vi "Main.vi"(8 "error in":errorcluster, 11 "TCP Server Example in":refnum<class "TCP Server Example.lvclass">) -> (0 "error out":errorcluster, 3 "TCP Server Example out":refnum<class "TCP Server Example.lvclass">)   [LabVIEW 2017, in "TCP Server Example.lvclass"]
doc: "The <b>Queued Message Handler</b> of the Worker that owns this VI."
uses:
  TCP Server Example.lvclass
  C:/SC/Source Code/VIPM/LabVIEW 20xx/vi.lib/addons/_Workers/Library/Classes/Worker/Worker.lvclass
  Client Data.ctl
  TCP Server Example.lvclass/TCP Server Example.ctl
  Initialization Data.ctl
  TCP Server/TCP Server/rqp_Start Listening.ctl
  TCP Server/TCP Server/rqp_Send String to Clients.ctl
  TCP Server/TCP Server/rqp_Disconnect Clients.ctl
  <vilib>/addons/_Workers/Library/Classes/Message Queue/Message Queue.lvclass
  TCP Server/TCP Server/TCP Server.lvclass
panel:
  in  "Server Name":string="TCP Server"
  out "Listening":bool
  in  "Server Port":u16=7654
  in  "Start/Stop Listening":bool caption="Disconnect from Server"
  in  "Client 2":T1
  out "Title":string="TCP Server Example"
  in  "Client 1":T1
  # "Server Name"
  # "Server Port"
  # "( 1 : N connections )"
  # "The Workers TCP Server can accept connections from multiple TCP Clients. This example shows how one TCP Server can be connected to two TCP Clients."
  # "Client Name :"
  # "IP Address :"
  # "Connected? :"
  # "Client Name :"
  # "IP Address :"
  # "Connected? :"
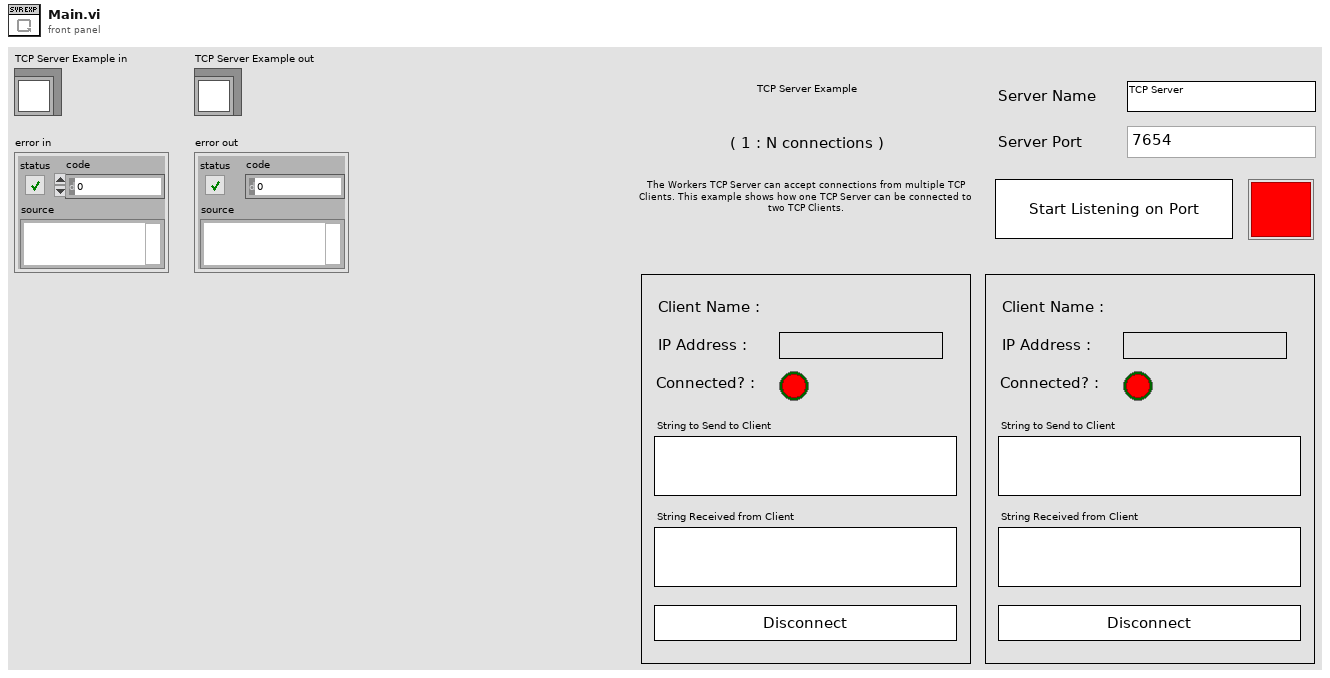
[diagram p1: front panel]
types:
  T1 = typedef "TCP Server Example.lvclass/Client Data.ctl" = cluster{"Client Name":string, "IP Address":string, "Connected?":bool, "String to Send to Client":string, "String Received from Client":string, "Disconnect from Client":bool}
  T2 = typedef "TCP Server Example.lvclass/Initialization Data.ctl" = cluster{"String":string}
  T3 = typedef "_TCP Server.lvlib/TCP Server.lvclass/rqp_Start Listening.ctl" = cluster{"Server Name":string, "Server IP Address":string, "Server Port":u16}
  T4 = typedef "_TCP Server.lvlib/TCP Server.lvclass/rqp_Send String to Clients.ctl" = cluster{"TCP Client Names":string[], "String to Send":string}
  T5 = typedef "_TCP Server.lvlib/TCP Server.lvclass/rqp_Disconnect Clients.ctl" = cluster{"TCP Client Names":string[]}
  T6 = typedef "_TCP Server.lvlib/TCP Server.lvclass/rsp_Connection Notify.ctl" = cluster{"Client Name":string, "IP Address":string, "Connected?":bool}
  T7 = typedef "_TCP Server.lvlib/TCP Server.lvclass/rsp_Incoming Data.ctl" = cluster{"Client Name":string, "Data":string}
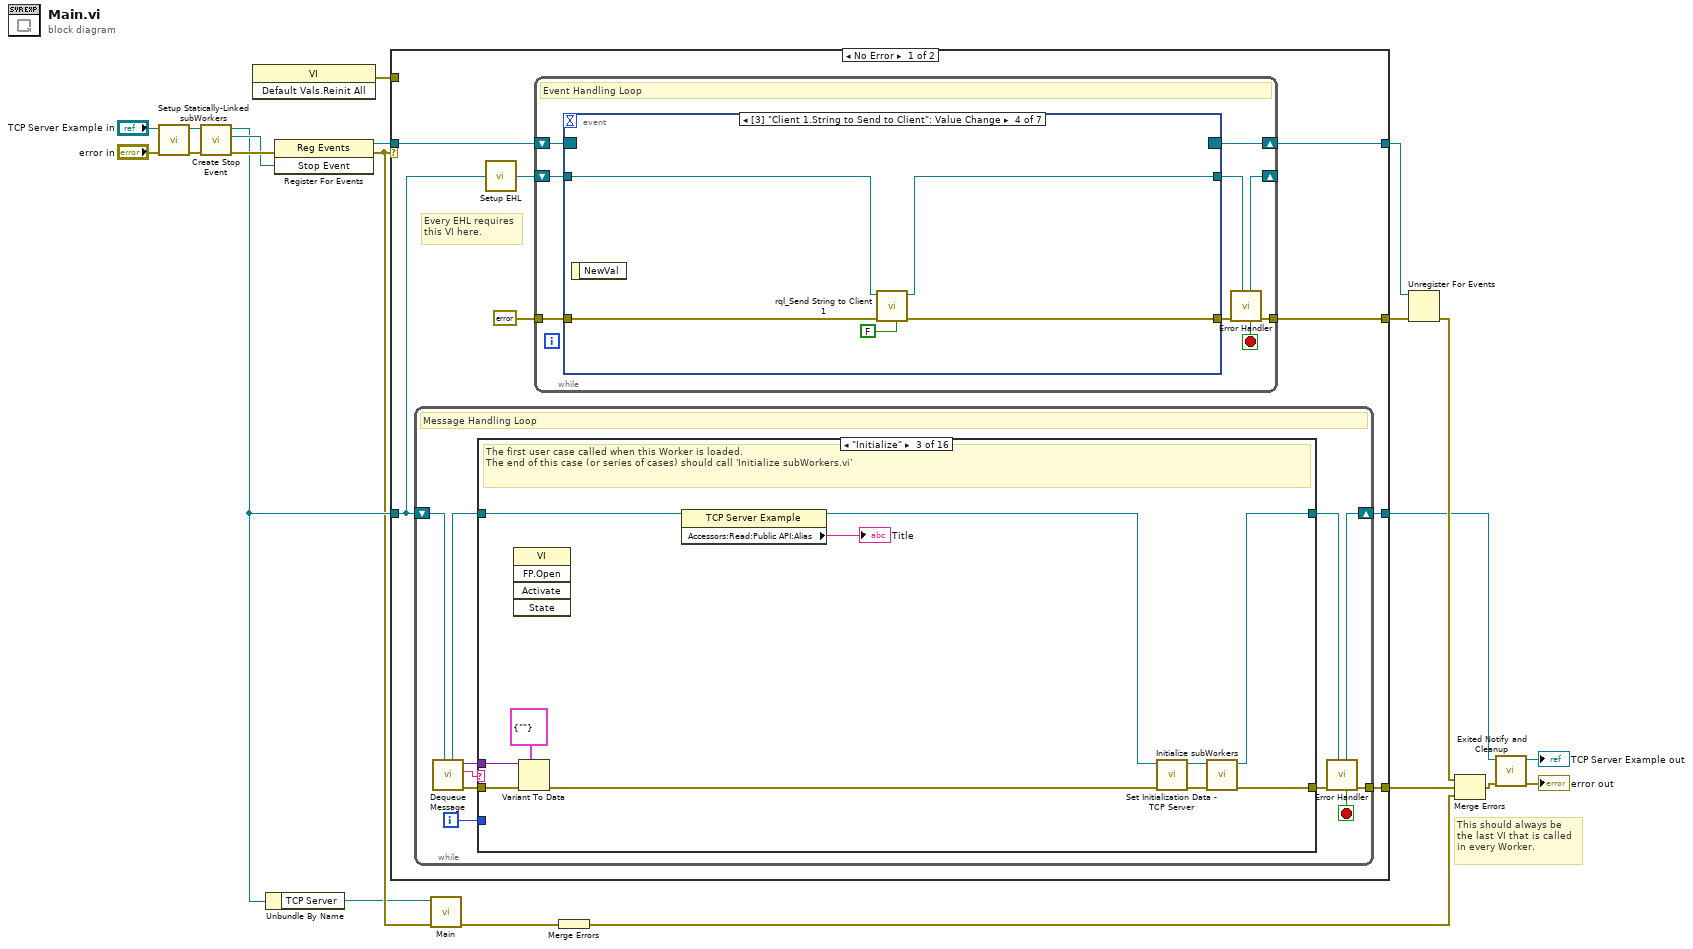
[diagram p0: block diagram]
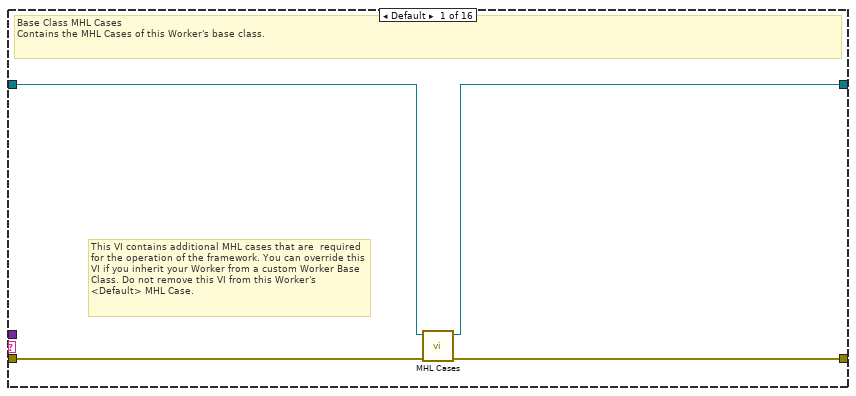
[diagram p2: hidden frame]
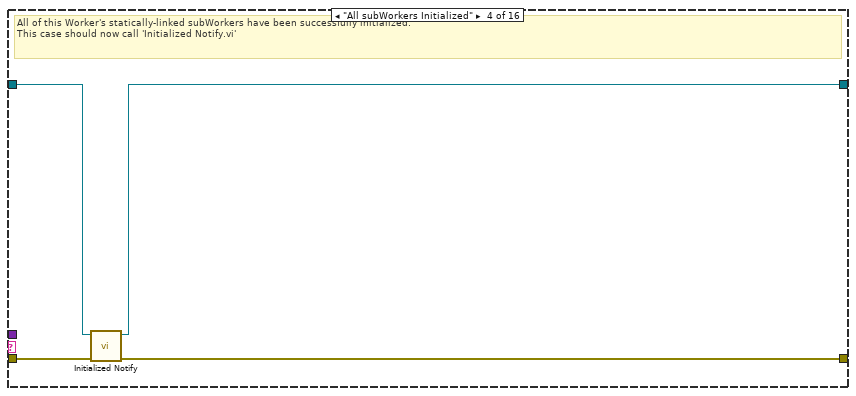
[diagram p4: hidden frame]
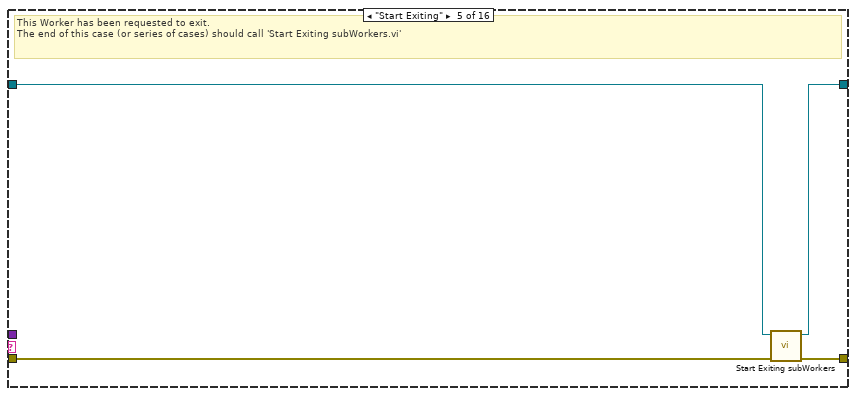
[diagram p5: hidden frame]
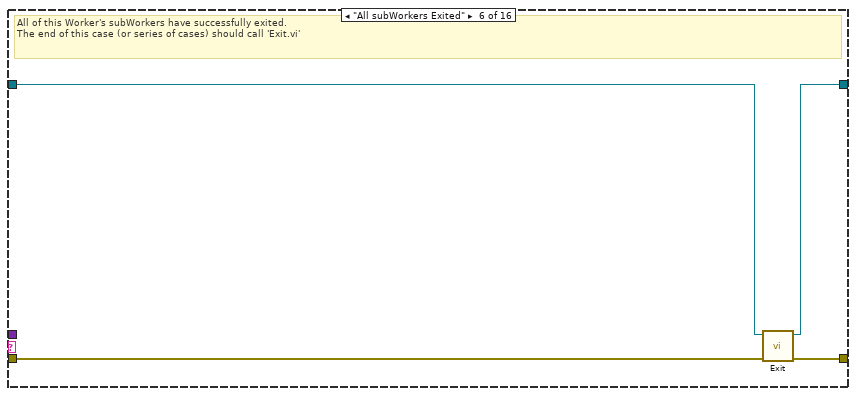
[diagram p6: hidden frame]
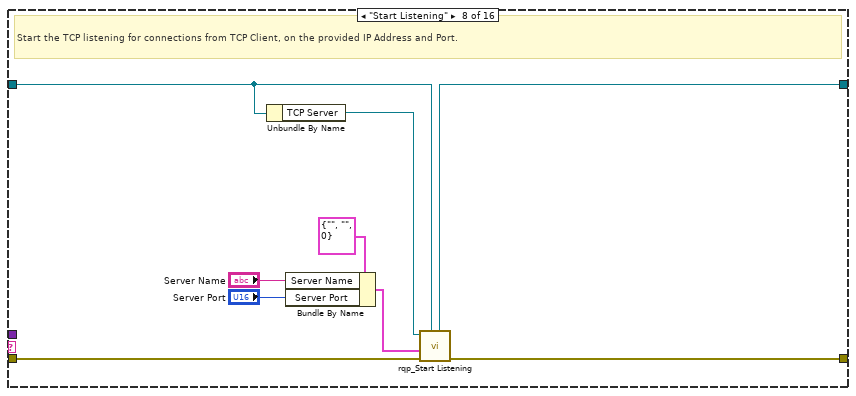
[diagram p8: hidden frame]
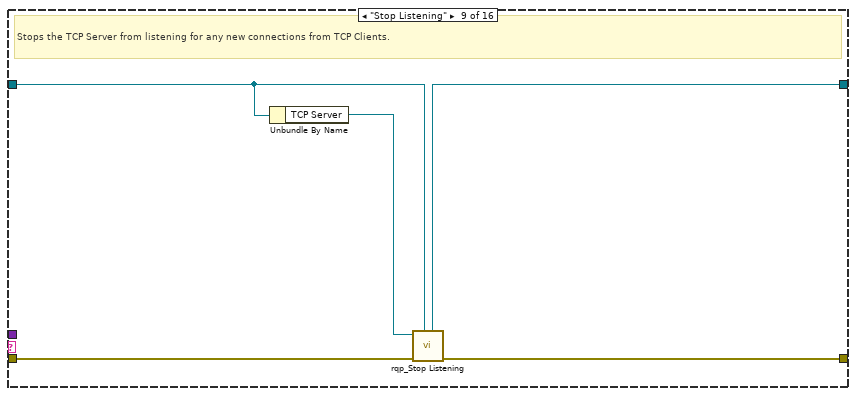
[diagram p9: hidden frame]
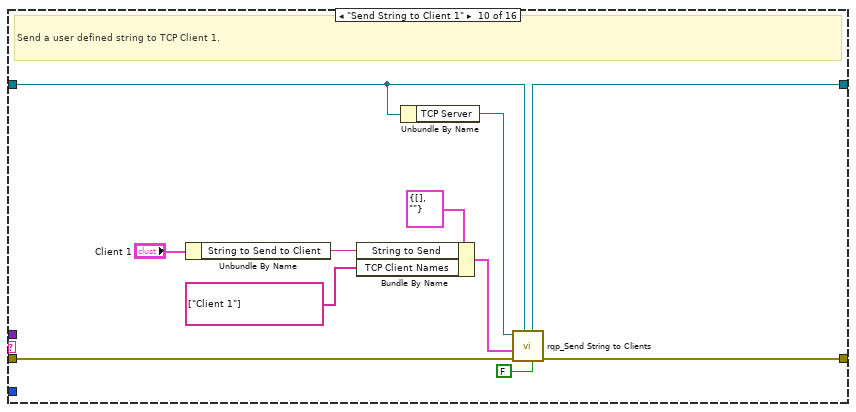
[diagram p10: hidden frame]
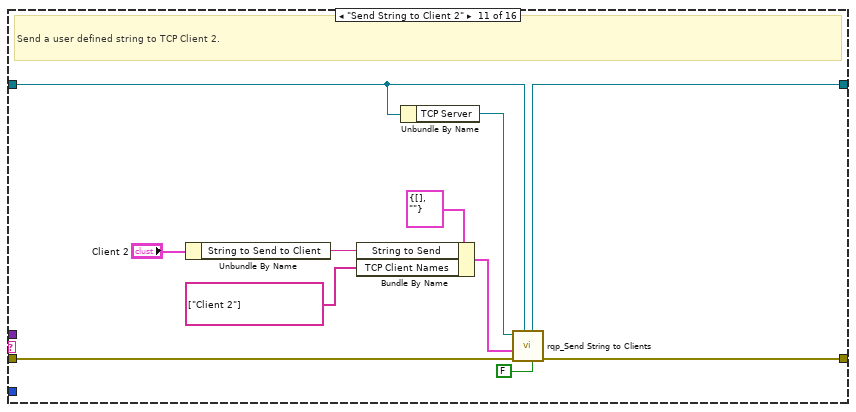
[diagram p11: hidden frame]
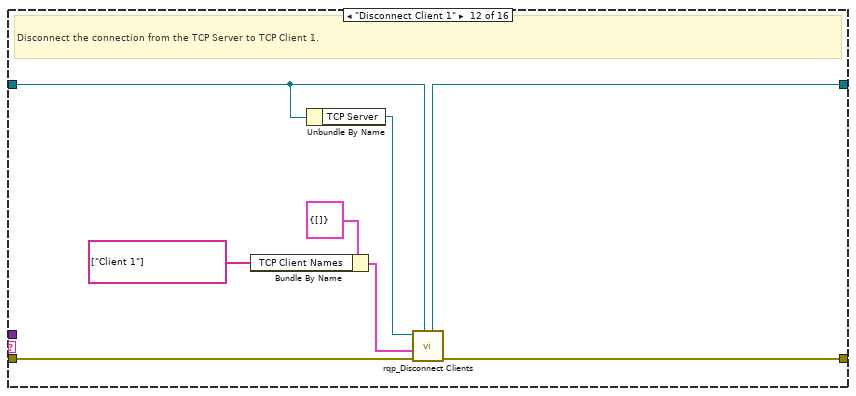
[diagram p12: hidden frame]
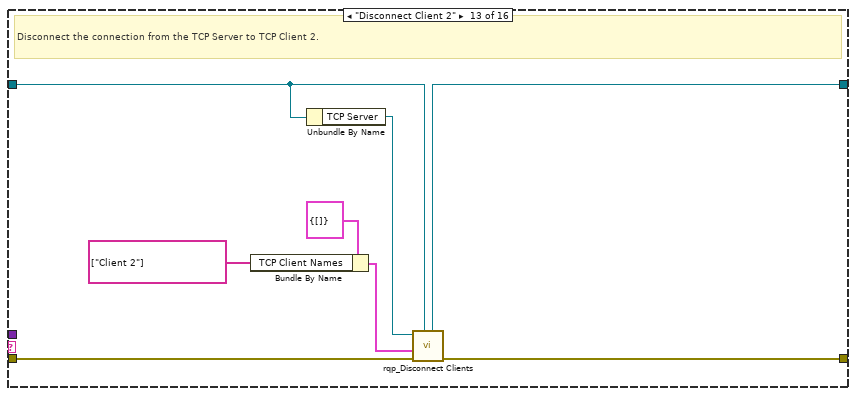
[diagram p13: hidden frame]
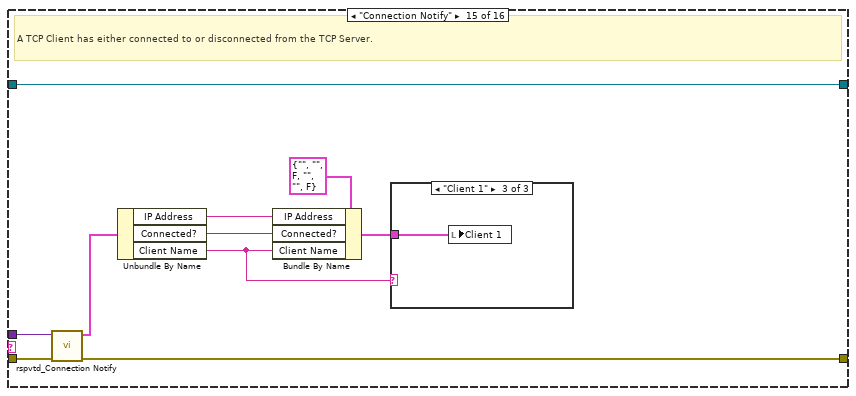
[diagram p15: hidden frame]
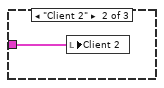
[diagram p17: hidden frame]
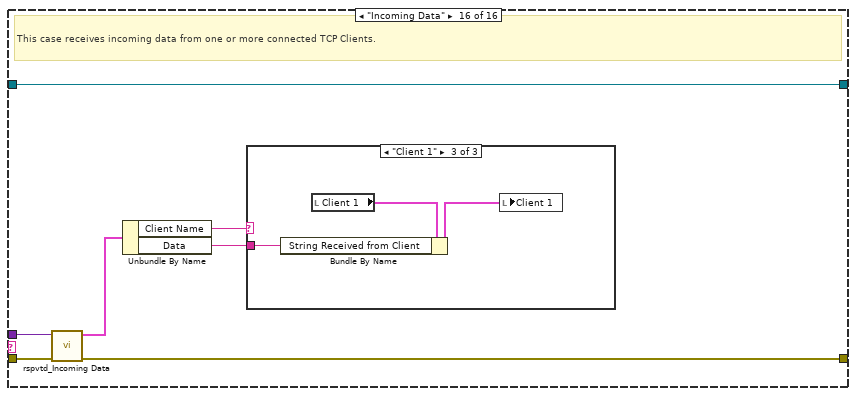
[diagram p18: hidden frame]
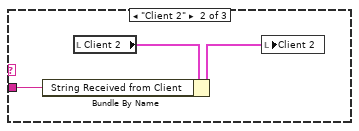
[diagram p20: hidden frame]
diagram:
  # "This should always be the last VI that is called in every Worker."
  n1 = call "Setup Statically-Linked subWorkers.vi"("error in"="error in", "TCP Server Example in"="TCP Server Example in") -> ("error out"=w6:errorcluster, "TCP Server Example out"=w4:refnum<class "TCP Server Example.lvclass">)  [unwired: 8 in]
  n2 = call-dynamic "Create Stop Event.vi"("error in"=w6, "Worker"=w4) -> ("error out"=w16:errorcluster, "Stop Event"=w13:refnum<user-event>, "Worker out"=w10:refnum<class "TCP Server Example.lvclass">)  [unwired: 7 in]
  n3 = invoke class="VI" method="Default Vals.Reinit All"() -> (error out=w8:errorcluster)  [unwired: 3 in, 2 out]
  n4 = Unbundle By Name(w10) -> ("TCP Server"=w1:refnum<class "TCP Server.lvclass">)
  n5 = register-events(error in=w16, w13) -> (reference out=w15:refnum<event-registration>, error out=w9:errorcluster)  [unwired: 1 in]
  n6 = case shown="No Error" w9 {
    tunnel: w10 -> [w24 w211]
    tunnel: [w22 w212] -> w14
    tunnel: w15 -> [w29 w213]
    tunnel: [w26 w214] -> w20
    tunnel: [w28 w213] -> w19
    tunnel: [w23 w210] -> w17
    selector: w9 -> [_ w214]
    tunnel: w8 -> [_ _]
    frame No Error {
      # "Every EHL requires\nthis VI here."
      n7 = while {
        shift-right: [w38] -> w23
        shift-left: w24 -> [w40]
        tunnel: [w39] -> w22
        i -> [w31]
        stop <- w32 stop-if-true
        # "Message Handling Loop"
        n8 = call-dynamic "Dequeue Message.vi"("Worker"=w40) -> ("error out"=w37:errorcluster, "Case out"=w33:string, "Data out"=w30:variant, "Worker out"=w35:refnum<class "TCP Server Example.lvclass">)  [unwired: 6 in, 1 out]
        n9 = case "Worker MHL Case Structure (DO NOT CHANGE LABEL NAME)" shown="\"Initialize\"" w33 {
          tunnel: w37 -> [w44 w45 w55 w60 w62 w69 w71 w80 w85 w96 w107 w115 w123 w125 w135 w144]
          tunnel: [w43 w45 w57 w58 w65 w68 w71 w79 w84 w95 w106 w114 w122 w125 w133 w142] -> w36
          tunnel: w35 -> [w42 w46 w52 w61 w63 w67 w70 w73 w82 w92 w104 w112 w120 w124 w134 w143]
          tunnel: [w41 w46 w56 w59 w64 w66 w70 w78 w83 w94 w105 w113 w121 w124 w134 w143] -> w34
          tunnel: w31 -> [_ _ _ _ _ _ _ _ _ _ _ _ _ _ _ _]
          tunnel: w30 -> [_ _ w53 _ _ _ _ _ _ _ _ _ _ _ w132 w141]
          frame Default {
            # "This VI contains additional MHL cases that are  required for the operation of the framework. You can override this VI if you inherit your Worker from a custom Worker Base Class. Do not remove this VI from this Worker's <Default> MHL Case."
            # "Base Class MHL Cases\nContains the MHL Cases of this Worker's base class."
            n10 = call-dynamic "MHL Cases.vi"("error in"=w44, "Worker in"=w42) -> ("error out"=w43:errorcluster, "Worker out"=w41:refnum<class "TCP Server Example.lvclass">)  [unwired: 8 in]
          }
          frame "------------ FRAMEWORK CASES -----------" {
            # "Start of Workers Framework Cases"
          }
          frame "Initialize" {
            # "The first user case called when this Worker is loaded.\nThe end of this case (or series of cases) should call 'Initialize subWorkers.vi'"
            n11 = invoke class="VI" method="FP.Open"() -> ()  [unwired: 5 in, 5 out]
            n12 = Variant To Data(error in=w55, type=T2 {"String"=""} ("Initialization Data"), Variant=w53) -> (error out=w54:errorcluster)  [unwired: 1 out]
            n13 = property class="TCP Server Example"(reference=w52) -> (reference out=w47:refnum<class "TCP Server Example.lvclass">, "Accessors:Read:Public API:Alias"=→"Title":string)  [unwired: 1 in, 1 out]
            n14 = call "Set Initialization Data - TCP Server.vi"("error in"=w54, "TCP Server Example in"=w47) -> ("error out"=w49:errorcluster, "TCP Server Example out"=w48:refnum<class "TCP Server Example.lvclass">)  [unwired: 8 in]
            n15 = call-dynamic "Initialize subWorkers.vi"("error in"=w49, "Worker"=w48) -> ("error out"=w57:errorcluster, "dup Worker out"=w56:refnum<class "TCP Server Example.lvclass">)  [unwired: 8 in]
          }
          frame "All subWorkers Initialized" {
            # "All of this Worker's statically-linked subWorkers have been successfully initialized.\nThis case should now call 'Initialized Notify.vi'"
            n16 = call-dynamic "Initialized Notify.vi"("error in"=w60, "Worker"=w61) -> ("error out"=w58:errorcluster, "dup Worker out"=w59:refnum<class "TCP Server Example.lvclass">)  [unwired: 8 in]
          }
          frame "Start Exiting" {
            # "This Worker has been requested to exit. \nThe end of this case (or series of cases) should call 'Start Exiting subWorkers.vi'"
            n17 = call-dynamic "Start Exiting subWorkers.vi"("error_in"=w62, "Worker"=w63) -> ("error out"=w65:errorcluster, "dup Worker out"=w64:refnum<class "TCP Server Example.lvclass">)  [unwired: 8 in]
          }
          frame "All subWorkers Exited" {
            # "All of this Worker's subWorkers have successfully exited. \nThe end of this case (or series of cases) should call 'Exit.vi'"
            n18 = call-dynamic "Exit.vi"("error_in"=w69, "Worker"=w67) -> ("error out"=w68:errorcluster, "dup Worker out"=w66:refnum<class "TCP Server Example.lvclass">)  [unwired: 8 in]
          }
          frame "------------- LOCAL API CASES -------------" {
            # "Start of Workers Local API Cases"
          }
          frame "Start Listening" {
            # "Start the TCP listening for connections from TCP Client, on the provided IP Address and Port."
            n19 = Unbundle By Name(w73) -> ("TCP Server"=w72:refnum<class "TCP Server.lvclass">)
            n20 = Bundle By Name(cluster=T3 {"Server Name"="", "Server IP Address"="", "Server Port"=0} ("Data"), "Server Name"="Server Name", "Server Port"="Server Port") -> (w76:T3)
            n21 = call "rqp_Start Listening.vi"("Caller in"=w73, "error in"=w80, "Data in"=w76, "TCP Server in"=w72) -> ("error out"=w79:errorcluster, "dup Caller out"=w78:refnum<class "TCP Server Example.lvclass">)  [unwired: 5 in, 1 out]
          }
          frame "Stop Listening" {
            # "Stops the TCP Server from listening for any new connections from TCP Clients."
            n22 = Unbundle By Name(w82) -> ("TCP Server"=w81:refnum<class "TCP Server.lvclass">)
            n23 = call "rqp_Stop Listening.vi"("Caller in"=w82, "error in"=w85, "TCP Server in"=w81) -> ("error out"=w84:errorcluster, "dup Caller out"=w83:refnum<class "TCP Server Example.lvclass">)  [unwired: 6 in, 1 out]
          }
          frame "Send String to Client 1" {
            # "Send a user defined string to TCP Client 1."
            n24 = Unbundle By Name("Client 1") -> ("String to Send to Client"=w88:string)
            n25 = Bundle By Name(cluster=T4 {"TCP Client Names"=[], "String to Send"=""} ("Data in"), "String to Send"=w88, "TCP Client Names"=string[] ["Client 1"]) -> (w89:T4)
            n26 = Unbundle By Name(w92) -> ("TCP Server"=w91:refnum<class "TCP Server.lvclass">)
            n27 = call "rqp_Send String to Clients.vi"("Show in Debugger?"=FALSE, "Caller in"=w92, "error in"=w96, "Data in"=w89, "TCP Server in"=w91) -> ("error out"=w95:errorcluster, "dup Caller out"=w94:refnum<class "TCP Server Example.lvclass">)  [unwired: 4 in, 1 out]
          }
          frame "Send String to Client 2" {
            # "Send a user defined string to TCP Client 2."
            n28 = Unbundle By Name("Client 2") -> ("String to Send to Client"=w100:string)
            n29 = Bundle By Name(cluster=T4 {"TCP Client Names"=[], "String to Send"=""} ("Data in"), "String to Send"=w100, "TCP Client Names"=string[] ["Client 2"]) -> (w101:T4)
            n30 = Unbundle By Name(w104) -> ("TCP Server"=w103:refnum<class "TCP Server.lvclass">)
            n31 = call "rqp_Send String to Clients.vi"("Show in Debugger?"=FALSE, "Caller in"=w104, "error in"=w107, "Data in"=w101, "TCP Server in"=w103) -> ("error out"=w106:errorcluster, "dup Caller out"=w105:refnum<class "TCP Server Example.lvclass">)  [unwired: 4 in, 1 out]
          }
          frame "Disconnect Client 1" {
            # "Disconnect the connection from the TCP Server to TCP Client 1."
            n32 = Bundle By Name(cluster=T5 {"TCP Client Names"=[]} ("Data in"), "TCP Client Names"=string[] ["Client 1"]) -> (w109:T5)
            n33 = Unbundle By Name(w112) -> ("TCP Server"=w111:refnum<class "TCP Server.lvclass">)
            n34 = call "rqp_Disconnect Clients.vi"("Caller in"=w112, "error in"=w115, "Data in"=w109, "TCP Server in"=w111) -> ("error out"=w114:errorcluster, "dup Caller out"=w113:refnum<class "TCP Server Example.lvclass">)  [unwired: 5 in, 1 out]
          }
          frame "Disconnect Client 2" {
            # "Disconnect the connection from the TCP Server to TCP Client 2."
            n35 = Bundle By Name(cluster=T5 {"TCP Client Names"=[]} ("Data in"), "TCP Client Names"=string[] ["Client 2"]) -> (w117:T5)
            n36 = Unbundle By Name(w120) -> ("TCP Server"=w119:refnum<class "TCP Server.lvclass">)
            n37 = call "rqp_Disconnect Clients.vi"("Caller in"=w120, "error in"=w123, "Data in"=w117, "TCP Server in"=w119) -> ("error out"=w122:errorcluster, "dup Caller out"=w121:refnum<class "TCP Server Example.lvclass">)  [unwired: 5 in, 1 out]
          }
          frame "------------- RESPONSE CASES --------------" {
            # "Start of Workers Response Cases"
          }
          frame "Connection Notify" {
            # "A TCP Client has either connected to or disconnected from the TCP Server."
            n38 = call "rspvtd_Connection Notify.vi"("error in"=w135, "Data in"=w132) -> ("error out"=w133:errorcluster, "Data out"=w131:T6)  [unwired: 8 in]
            n39 = Unbundle By Name(w131) -> ("IP Address"=w128:string, "Connected?"=w129:bool, "Client Name"=w127:string)
            n40 = Bundle By Name(cluster=T1 {"Client Name"="", "IP Address"="", "Connected?"=FALSE, "String to Send to Client"="", "String Received from Client"="", "Disconnect from Client"=FALSE} ("Client Connection 1"), "IP Address"=w128, "Connected?"=w129, "Client Name"=w127) -> (w126:T1)
            n41 = case shown="\"Client 1\"" w127 {
              tunnel: w126 -> [_ w136 w137]
              frame Default {
              }
              frame "Client 2" {
                n42 = local write "Client 2"(w136) -> ()
              }
              frame "Client 1" {
                n43 = local write "Client 1"(w137) -> ()
              }
            }
          }
          frame "Incoming Data" {
            # "This case receives incoming data from one or more connected TCP Clients."
            n44 = call "rspvtd_Incoming Data.vi"("error in"=w144, "Data in"=w141) -> ("error out"=w142:errorcluster, "Data out"=w140:T7)  [unwired: 8 in]
            n45 = Unbundle By Name(w140) -> ("Client Name"=w139:string, "Data"=w138:string)
            n46 = case shown="\"Client 1\"" w139 {
              tunnel: w138 -> [_ w145 w148]
              frame Default {
              }
              frame "Client 2" {
                n47 = local read "Client 2"() -> (w147:T1)
                n48 = Bundle By Name(cluster=w147, "String Received from Client"=w145) -> (w146:T1)
                n49 = local write "Client 2"(w146) -> ()
              }
              frame "Client 1" {
                n50 = local read "Client 1"() -> (w150:T1)
                n51 = Bundle By Name(cluster=w150, "String Received from Client"=w148) -> (w149:T1)
                n52 = local write "Client 1"(w149) -> ()
              }
            }
          }
        }
        n53 = call-dynamic "Error Handler.vi"("Worker"=w34, "error_in"=w36) -> ("error out"=w39:errorcluster, "Stop Loop"=w32:bool, "Worker out"=w38:refnum<class "TCP Server Example.lvclass">)  [unwired: 7 in]
      }
      n54 = call-dynamic "Setup EHL.vi"("Worker"=w24) -> ("Worker out"=w25:refnum<class "TCP Server Example.lvclass">)  [unwired: 14 in]
      n55 = while "Event Handling Loop" {
        shift-right: [w159] -> w28
        shift-left: w29 -> [w158]
        tunnel: [w154] -> w26
        tunnel: errorcluster {"status"=FALSE, "code"=0, "source"=""} ("error constant") -> [w156]
        shift-right: [w152] -> _
        shift-left: w25 -> [w157]
        stop <- w151 stop-if-true
        # "Event Handling Loop"
        n56 = event shown="[3] \"Client 1.String to Send to Client\": Value Change" {
          selector: w158 -> [_ _ _ _ _ _ _]
          dyn-events: [_ _ _ _ _ _ _] -> w159
          timeout: _ -> [_ _ _ _ _ _ _]
          tunnel: [w163 w170 w175 w189 w194 w198 w205] -> w155
          tunnel: w156 -> [w164 w169 w177 w190 w195 w202 w209]
          tunnel: w157 -> [w162 w168 w174 w188 w193 w197 w204]
          tunnel: [w161 w167 w173 w187 w192 w196 w203] -> w153
          event User Event {
            # "EHL Stop Event. This EHL exits from this case."
            n57 = event-data() -> ("Stop Event Data"=w160:variant)  [unwired: 1 in]
            n58 = call-dynamic "EHL Stop - EHL Case.vi"("error in"=w164, "Stop Event Data"=w160, "Worker"=w162) -> ("error out"=w163:errorcluster, "Worker out"=w161:refnum<class "TCP Server Example.lvclass">)  [unwired: 7 in]
          }
          event Panel Close? {
            # "Calls the Start Exiting case of this Worker. This will start the exiting sequence of this Worker."
            n59 = event-data() -> ()  [unwired: 1 in, 1 out]
            n60 = property class="TCP Server Example"(reference=w168) -> (reference out=w166:refnum<class "TCP Server Example.lvclass">, "Accessors:Read:Public API:Queue"=w165:refnum<class "Message Queue.lvclass">)  [unwired: 1 in, 1 out]
            n61 = call-dynamic "Worker Start Exiting.vi"("error_in"=w169, "Message Queue"=w165, "Worker"=w166) -> ("error out"=w170:errorcluster, "dup Worker out"=w167:refnum<class "TCP Server Example.lvclass">)  [unwired: 7 in]
            n62 = event-data ("Event Filter Node")("Discard?"=TRUE) -> ()  [unwired: 1 in, 1 out]
          }
          event "Start/Stop Listening": Value Change {
            n63 = event-data() -> ("NewVal"=w172:bool)  [unwired: 1 in]
            n64 = case shown="True" w172 {
              tunnel: w177 -> [w181 w185]
              tunnel: [w180 w184] -> w175
              tunnel: w174 -> [w179 w183]
              tunnel: [w178 w182] -> w173
              frame True {
                n65 = call "rql_Start Listening.vi"("error in"=w181, "TCP Server Example in"=w179) -> ("error out"=w180:errorcluster, "dup TCP Server Example out"=w178:refnum<class "TCP Server Example.lvclass">)  [unwired: 8 in]
              }
              frame False {
                n66 = call "rql_Stop Listening.vi"("error in"=w185, "TCP Server Example in"=w183) -> ("error out"=w184:errorcluster, "dup TCP Server Example out"=w182:refnum<class "TCP Server Example.lvclass">)  [unwired: 8 in]
              }
            }
            "Listening" <- "Start/Stop Listening"
          }
          event Value Change {
            n67 = event-data() -> ()  [unwired: 1 in, 1 out]
            n68 = call "rql_Send String to Client 1.vi"("Show in Debugger?"=FALSE, "error in"=w190, "TCP Server Example in"=w188) -> ("error out"=w189:errorcluster, "dup TCP Server Example out"=w187:refnum<class "TCP Server Example.lvclass">)  [unwired: 7 in]
          }
          event Value Change {
            n69 = event-data() -> ()  [unwired: 1 in, 1 out]
            n70 = call "rql_Send String to Client 2.vi"("Show in Debugger?"=FALSE, "error in"=w195, "TCP Server Example in"=w193) -> ("error out"=w194:errorcluster, "dup TCP Server Example out"=w192:refnum<class "TCP Server Example.lvclass">)  [unwired: 7 in]
          }
          event Value Change {
            n71 = event-data() -> ()  [unwired: 1 in, 1 out]
            n72 = call "rql_Disconnect Client 1.vi"("error in"=w202, "TCP Server Example in"=w197) -> ("error out"=w198:errorcluster, "dup TCP Server Example out"=w196:refnum<class "TCP Server Example.lvclass">)  [unwired: 8 in]
            n73 = local read "Client 1"() -> (w199:T1)
            n74 = Bundle By Name(cluster=w199, "Disconnect from Client"=FALSE ("Connected?")) -> (w201:T1)
            n75 = local write "Client 1"(w201) -> ()
          }
          event Value Change {
            n76 = event-data() -> ()  [unwired: 1 in, 1 out]
            n77 = call "rql_Disconnect Client 2.vi"("error in"=w209, "TCP Server Example in"=w204) -> ("error out"=w205:errorcluster, "dup TCP Server Example out"=w203:refnum<class "TCP Server Example.lvclass">)  [unwired: 8 in]
            n78 = local read "Client 2"() -> (w206:T1)
            n79 = Bundle By Name(cluster=w206, "Disconnect from Client"=FALSE ("Connected?")) -> (w208:T1)
            n80 = local write "Client 2"(w208) -> ()
          }
        }
        n81 = call-dynamic "Error Handler.vi"("Worker"=w153, "error_in"=w155) -> ("error out"=w154:errorcluster, "Stop Loop"=w151:bool, "Worker out"=w152:refnum<class "TCP Server Example.lvclass">)  [unwired: 7 in]
      }
    }
    frame Error {
      n82 = call-dynamic "Error Handler.vi"("Worker"=w211, "error_in"=w214) -> ("error out"=w212:errorcluster, "Worker out"=w210:refnum<class "TCP Server Example.lvclass">)  [unwired: 7 in, 1 out]
    }
  }
  n83 = call-dynamic "Main.vi"("error in"=w9, "TCP Server in"=w1) -> ("error out"=w3:errorcluster)  [unwired: 8 in, 1 out]
  n84 = Merge Errors(w3) -> (w2:errorcluster)
  n85 = Unregister For Events(event registration refnum=w19, error in=w20) -> (error out=w21:errorcluster)
  n86 = Merge Errors(w21, w14, w2) -> (w18:errorcluster)
  n87 = call-dynamic "Exited Notify and Cleanup.vi"("error_in"=w18, "Worker"=w17) -> ("error out"=→"error out":errorcluster, "dup Worker out"=→"TCP Server Example out":refnum<class "TCP Server Example.lvclass">)  [unwired: 8 in]
